vi "FFT Filter.vi"(8 "error in":errorcluster, 10 "Channel in":refnum<class "Producer Channel.lvclass">, 11 "Data in":dbl[](array[numeric])) -> (0 "error out":errorcluster, 3 "Data out":dbl[](array[numeric]))   [LabVIEW 2024, in "FFT.lvlib" / "FFT.lvclass"]
uses:
  FFT.lvclass
  <vilib>/FlexLogger/SDK/PluginSDK.lvlibp/PEFClasses/SDK/Producer Channel/Producer Channel.lvclass
  <vilib>/Analysis/3filter.llb/Filter Passband Type.ctl
  <vilib>/Analysis/3filter.llb/Butterworth Filter (DBL).vi
  <vilib>/Analysis/NI_AALBase.lvlib
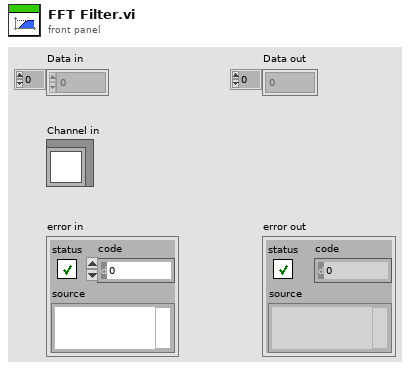
[diagram p1: front panel]
types:
  T1 = typedef "NI_AALBase.lvlib/Filter Passband Type.ctl" = enum32{"Lowpass", "Highpass", "Bandpass", "Bandstop"}
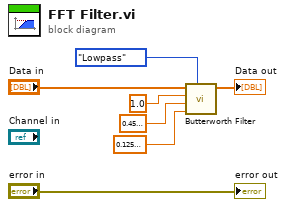
[diagram p0: block diagram]
diagram:
  n1 = call-poly <vilib>:"Butterworth Filter.vi"("filter type"=Filter_Passband_Type."Lowpass", "low cutoff freq: fl"=0.12500000000000006, "high cutoff freq: fh"=0.45000000000000007, "sampling freq: fs"=1.0, "X"="Data in") -> ("Filtered X"=→"Data out":dbl[])  [unwired: 3 in, 1 out]
  "error out" <- "error in"
